vi "KE2260B Get Display Text.vi"(8 "error in (no error)":errorcluster, 11 "VISA resource name":refnum<visa-resource-name>) -> (0 "error out":errorcluster, 1 "Text count":u32, 2 "Display Text":string, 3 "VISA resource name out":refnum<visa-resource-name>, 4 "Display Blink":bool)   [LabVIEW 2009, in "Keithley 2260B.lvlib"]
doc: "Returns display text and blink status."
uses:
  <instrlib>/Keithley 2260B/Keithley 2260B.lvlib
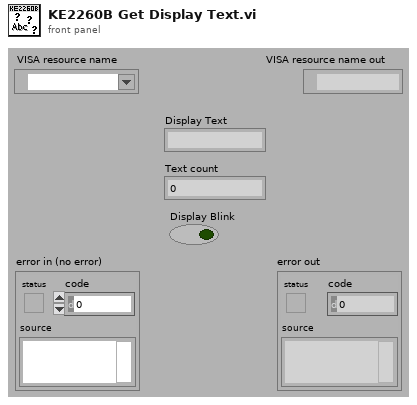
[diagram p1: front panel]
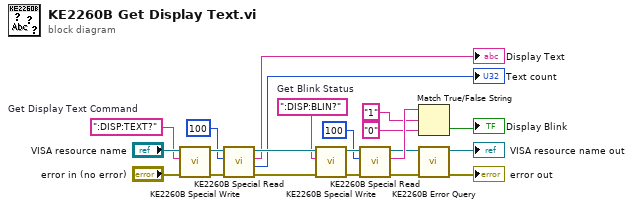
[diagram p0: block diagram]
diagram:
  w5 = ":DISP:TEXT?"  # Get Display Text Command
  w4 = ":DISP:BLIN?"  # Get Blink Status
  n1 = call <instrlib>:"KE2260B Special Write.vi"("error in (no error)"="error in (no error)", "Write Buffer (\"\")"=w5, "VISA session"="VISA resource name") -> ("error out"=w17:errorcluster, "dup VISA session"=w18:refnum<visa-resource-name>)  [unwired: 6 in, 1 out]
  n2 = call <instrlib>:"KE2260B Special Read.vi"("error in (no error)"=w17, "byte count"=u32 100, "VISA session"=w18) -> ("error out"=w8:errorcluster, "Return Count"=→"Text count":u32, "read buffer"=→"Display Text":string, "dup VISA session"=w9:refnum<visa-resource-name>)  [unwired: 5 in]
  n3 = call <instrlib>:"KE2260B Special Write.vi"("error in (no error)"=w8, "Write Buffer (\"\")"=w4, "VISA session"=w9) -> ("error out"=w11:errorcluster, "dup VISA session"=w12:refnum<visa-resource-name>)  [unwired: 6 in, 1 out]
  n4 = call <instrlib>:"KE2260B Special Read.vi"("error in (no error)"=w11, "byte count"=u32 100, "VISA session"=w12) -> ("error out"=w6:errorcluster, "read buffer"=w15:string, "dup VISA session"=w7:refnum<visa-resource-name>)  [unwired: 5 in, 1 out]
  n5 = Match True/False String(2:"0" ("false string"), 3:"1" ("true string"), 4:w15) -> (0:→"Display Blink":bool)  [unwired: 1 out]
  n6 = call <instrlib>:"KE2260B Error Query.vi"("error in (no error)"=w6, "VISA resource name"=w7) -> ("error out"=→"error out":errorcluster, "VISA resource name out"=→"VISA resource name out":refnum<visa-resource-name>)  [unwired: 6 in, 2 out]
